vi "清除波形.vi"(1 "板子选择":bool) -> (0 "输出字符串":string)   [LabVIEW 2017]
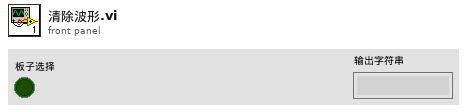
[diagram p1: front panel]
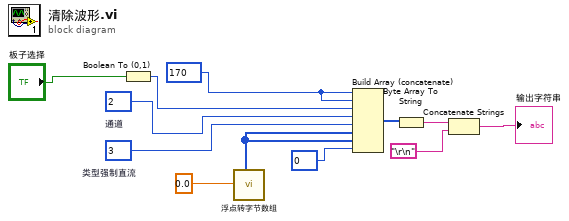
[diagram p0: block diagram]
diagram:
  w6 = 3  # 类型强制直流
  w10 = 2  # 通道
  w12 = 170
  n1 = Boolean To (0,1)(Boolean="板子选择") -> (0, 1=w5:i16)
  n2 = call "浮点转字节数组.vi"("输入"=0.0) -> ("数组，高字节在前"=w8:u8[])  [unwired: 3 in, 4 out]
  n3 = Build Array (concatenate)(w12, w12, w5, w10, w6, w8, w8, 0) -> (w11:i32[])
  n4 = Byte Array To String(unsigned byte array=w11) -> (string=w3:string)
  n5 = Concatenate Strings(w3, "\r\n") -> (→"输出字符串":string)
